vi "trace_property_double_sub.vi"(5 "trace idx global":u32, 7 "properties ui":string[](array[string]), 11 "error in (no error)":errorcluster) -> (8 "property":cluster{"property":string, "property value":dbl}, 10 "properties":T1(array[cluster]), 15 "error out":errorcluster)   [LabVIEW 2010, in "OSA.lvclass"]
uses:
  OSA.lvclass
  FTSLib.dll
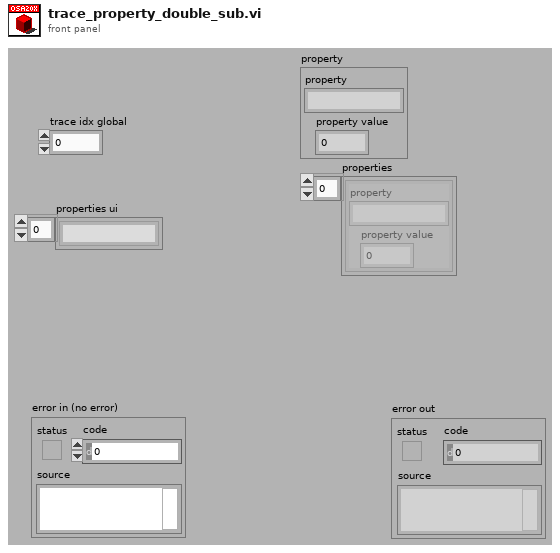
[diagram p1: front panel]
types:
  T1 = cluster{"property":string, "property value":dbl}[]
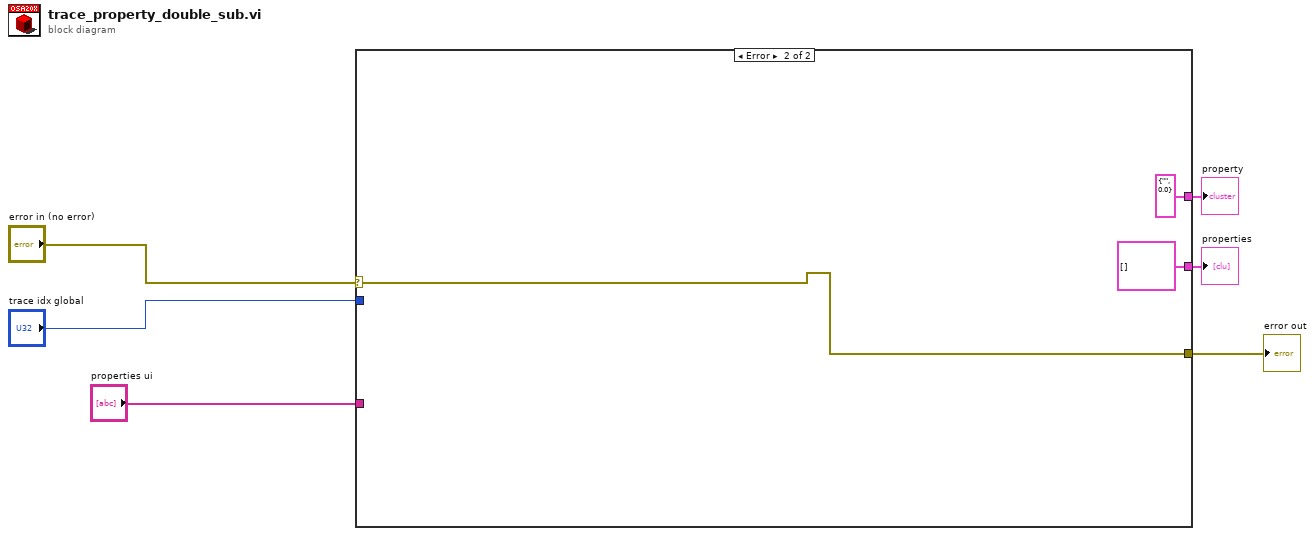
[diagram p0: block diagram]
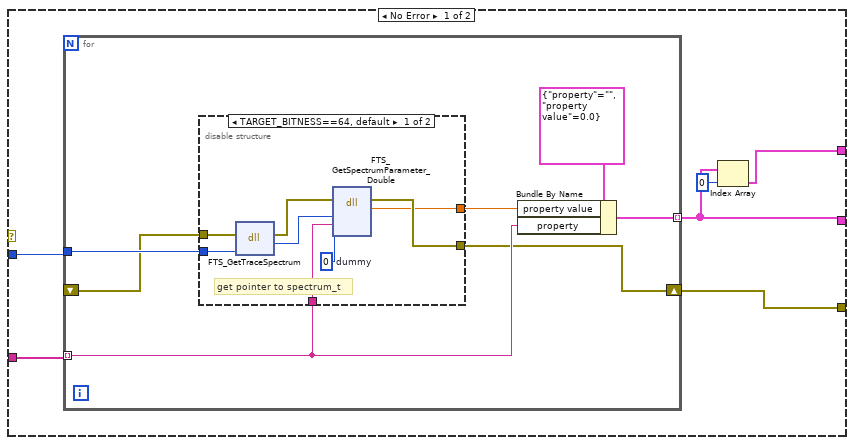
[diagram p2: hidden frame]
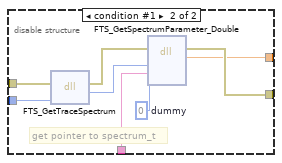
[diagram p3: hidden frame]
diagram:
  n1 = case shown="Error" "error in (no error)" {
    selector: "error in (no error)" -> [_ w38]
    tunnel: "properties ui" -> [w11 _]
    tunnel: "trace idx global" -> [w12 _]
    tunnel: [w8 T1 []] -> w1
    tunnel: [w10 cluster{"property":string, "property value":dbl} {"property"="", "property value"=0.0}] -> w2
    tunnel: [w7 w38] -> w4
    frame No Error {
      n2 = for {
        tunnel: w12 -> [w19]
        shift-right: [w14] -> w7
        shift-left: _ -> [w18]
        tunnel: w11 -> [w17] mode=indexing
        tunnel: [w13] -> w8 mode=indexing
        n3 = disable-structure shown="TARGET_BITNESS==64, default" {
          disable-tunnel: w19 -> [w27 w31]
          disable-tunnel: w17 -> [w26 w30]
          disable-tunnel: w18 -> [w23 w32]
          disable-tunnel: [w22 w29] -> w14
          disable-tunnel: [w21 w28] -> w15
          frame condition #0 (active) {
            w20 = u32 0  # dummy
            # "get pointer to spectrum_t"
            n4 = dll-call lib="FTSLib.dll" fn="FTS_GetTraceSpectrum"(error in=w23, "traceIdx"=w27) -> (error out=w24:errorcluster, "spectrum_t_pointer"=w25:u64)  [unwired: 3 in, 1 out]
            n5 = dll-call lib="FTSLib.dll" fn="FTS_GetSpectrumParameter_Double"(error in=w24, "spectrum_t_pointer"=w25, "parameter_name"=w26, "array_index"=w20) -> (error out=w22:errorcluster, "parameter"=w21:dbl)  [unwired: 5 in, 1 out]
          }
          frame condition #1 {
            w33 = u32 0  # dummy
            # "get pointer to spectrum_t"
            n6 = dll-call lib="FTSLib.dll" fn="FTS_GetTraceSpectrum"(error in=w32, "traceIdx"=w31) -> (error out=w34:errorcluster, "spectrum_t_pointer"=w35:u32)  [unwired: 3 in, 1 out]
            n7 = dll-call lib="FTSLib.dll" fn="FTS_GetSpectrumParameter_Double"(error in=w34, "spectrum_t_pointer"=w35, "parameter_name"=w30, "array_index"=w33) -> (error out=w29:errorcluster, "parameter"=w28:dbl)  [unwired: 5 in, 1 out]
          }
        }
        n8 = Bundle By Name(cluster=cluster{"property":string, "property value":dbl} {"property"="", "property value"=0.0}, "property value"=w15, "property"=w17) -> (w13:cluster{"property":string, "property value":dbl})
      }
      n9 = Index Array(array=w8, index=0) -> (element=w10:cluster{"property":string, "property value":dbl})
    }
    frame Error {
    }
  }
  "error out" <- w4
  "property" <- w2
  "properties" <- w1
